vi "s_interp.vi"(4 "Cluster":cluster{"Uin":dbl[][]}, 6 "Array 2":i16[](array[numeric])) -> (1 "Array":sgl[](array[numeric]))   [LabVIEW 2010]
uses:
  <vilib>/Analysis/NI_AALPro.lvlib
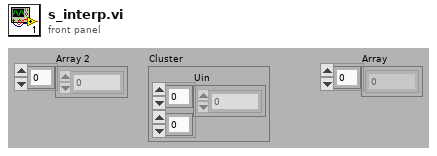
[diagram p1: front panel]
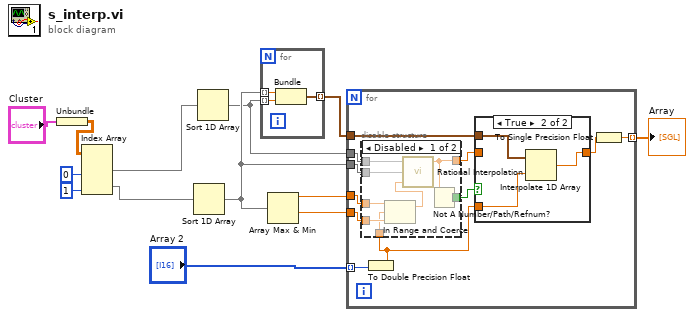
[diagram p0: block diagram]
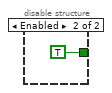
[diagram p2: hidden frame]
diagram:
  n1 = Unbundle("Cluster") -> ("Uin"=w5:dbl[][])
  n2 = Index Array(array=w5, index (col) #1=0 ("disabled index (col)"), index (col) #2=1 ("index (col)")) -> (element #1=w2:dbl[], element #2=w1:dbl[])  [unwired: 2 in]
  n3 = Sort 1D Array(array=w1) -> (sorted array=w7:dbl[])
  n4 = Sort 1D Array(array=w2) -> (sorted array=w6:dbl[])
  n5 = for {
    tunnel: w7 -> [w14] mode=indexing
    tunnel: w6 -> [w15] mode=indexing
    tunnel: [w16] -> w8 mode=indexing
    n6 = Bundle(w14, w15) -> (w16:cluster{dbl, dbl})  [unwired: 1 in]
  }
  n7 = Array Max & Min(array=w7) -> (max value=w12:dbl, min value=w13:dbl)  [unwired: 2 out]
  n8 = for {
    tunnel: "Array 2" -> [w26] mode=indexing
    tunnel: [w27] -> w10 mode=indexing
    tunnel: w6 -> [w25]
    tunnel: w7 -> [w24]
    tunnel: w12 -> [w23]
    tunnel: w13 -> [w22]
    tunnel: w8 -> [w20]
    n9 = To Double Precision Float(number=w26) -> (double precision float=w19:dbl)
    n10 = disable-structure shown="Disabled" {
      disable-tunnel: w25 -> [w34 _]
      disable-tunnel: w24 -> [w33 _]
      disable-tunnel: w23 -> [w32 _]
      disable-tunnel: w22 -> [w31 _]
      disable-tunnel: w19 -> [w30 _]
      disable-tunnel: [w29 _] -> w18
      disable-tunnel: [w28 TRUE] -> w17
      frame Disabled {
        n11 = In Range and Coerce(upper limit=w32, x=w30, lower limit=w31) -> (coerced(x)=w35:dbl)  [unwired: 1 out]
        n12 = call <vilib>:"Rational Interpolation.vi"("x value"=w35, "X"=w33, "Y"=w34) -> ("interpolation value"=w29:dbl)  [unwired: 2 out]
        n13 = Not A Number/Path/Refnum?(number/path/refnum=w29) -> (NaN/Path/Refnum?=w28:bool)
      }
      frame Enabled {
      }
    }
    n14 = case shown="True" w17 {
      tunnel: [w37 w38] -> w21
      tunnel: w18 -> [w37 _]
      tunnel: w20 -> [_ w40]
      tunnel: w19 -> [_ w39]
      frame False {
      }
      frame True {
        n15 = Interpolate 1D Array(1:w39, 2:w40) -> (0:w38:dbl)
      }
    }
    n16 = To Single Precision Float(number=w21) -> (single precision float=w27:sgl)
  }
  "Array" <- w10
